vi "Triangular PDF.vi"(8 "xmax":dbl=1.0, 9 "xmode":dbl=nan, 10 "xmin":dbl, 11 "x":dbl=0.5) -> (0 "error":i32, 3 "pdf(x)":dbl=2.0)   [LabVIEW 2018, in "NI_Gmath.lvlib"]
doc: "Computes the continuous probability density function (PDF) of various distributions. You must manually select the polymorphic instance to use."
uses:
  NI_Gmath.lvlib
  st_error_code.ctl
panel:
  # "Triangular PDF"
  # "NaN maps to \n(xmax-xmin)/2"
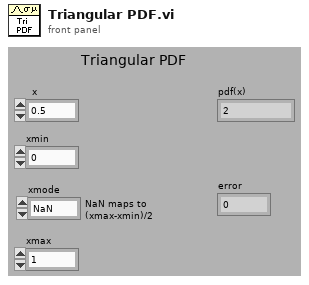
[diagram p1: front panel]
types:
  T1 = typedef "NI_Gmath.lvlib/st_error_code.ctl" = i32
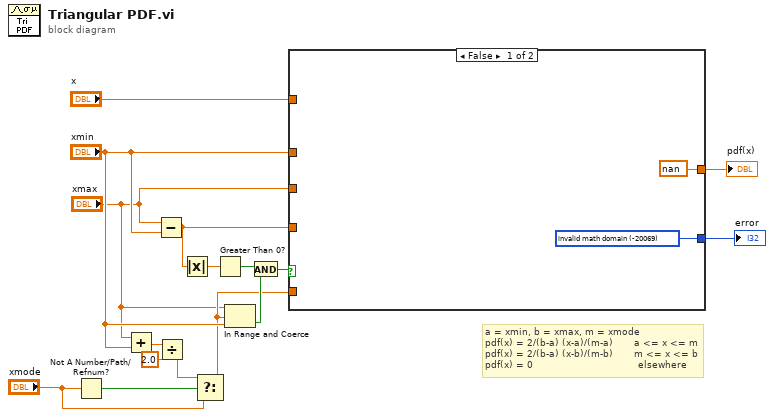
[diagram p0: block diagram]
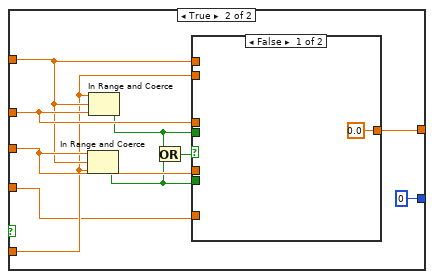
[diagram p2: hidden frame]
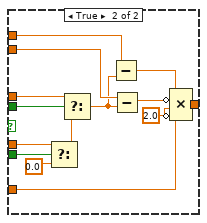
[diagram p3: hidden frame]
diagram:
  # "a = xmin, b = xmax, m = xmode\npdf(x) = 2/(b-a) (x-a)/(m-a)       a <= x <= m\npdf(x) = 2/(b-a) (x-b)/(m-b)       m <= x <= b\npdf(x) = 0                                   elsewhere"
  n1 = Not A Number/Path/Refnum?(number/path/refnum="xmode") -> (NaN/Path/Refnum?=w5:bool)
  n2 = Add(x="xmax", y="xmin") -> (x+y=w8:dbl)
  n3 = Subtract(x="xmax", y="xmin") -> (x-y=w10:dbl)
  n4 = Divide(x=w8, y=2.0) -> (x/y=w6:dbl)
  n5 = Absolute Value(x=w10) -> (abs(x)=w15:dbl)
  n6 = Select(t=w6, s=w5, f="xmode") -> (s? t:f=w2:dbl)
  n7 = Greater Than 0?(x=w15) -> (x > 0?=w12:bool)
  n8 = In Range and Coerce(upper limit="xmax", x=w2, lower limit="xmin") -> (In Range?=w3:bool)  [unwired: 1 out]
  n9 = And(x=w12, y=w3) -> (x .and. y?=w11:bool)
  n10 = case shown="False" w11 {
    tunnel: "x" -> [_ w25]
    tunnel: "xmin" -> [_ w27]
    tunnel: w10 -> [_ w23]
    tunnel: [nan w22] -> w14
    tunnel: [w17 0] -> w13
    tunnel: w2 -> [_ w24]
    tunnel: "xmax" -> [_ w26]
    frame False {
      w17 = T1 -20069 items=["invalid math domain"=-20069, "Fourier interpolation size m >= n"=-20070, "empty array"=-20003] ("stat interp error code")
    }
    frame True {
      n11 = In Range and Coerce(upper limit=w26, x=w25, lower limit=w24) -> (In Range?=w20:bool)  [unwired: 1 out]
      n12 = In Range and Coerce(upper limit=w24, x=w25, lower limit=w27) -> (In Range?=w21:bool)  [unwired: 1 out]
      n13 = Or(x=w21, y=w20) -> (x .or. y?=w19:bool)
      n14 = case shown="False" w19 {
        tunnel: w21 -> [_ w43]
        tunnel: w27 -> [_ w42]
        tunnel: w20 -> [_ w41]
        tunnel: w26 -> [_ w40]
        tunnel: w25 -> [_ w37]
        tunnel: w24 -> [_ w36]
        tunnel: w23 -> [_ w31]
        tunnel: [0.0 w30] -> w22
        frame False {
        }
        frame True {
          n15 = Select(t=w40, s=w41, f=0.0) -> (s? t:f=w39:dbl)
          n16 = Select(t=w42, s=w43, f=w39) -> (s? t:f=w35:dbl)
          n17 = Subtract(x=w37, y=w35) -> (x-y=w34:dbl)
          n18 = Subtract(x=w36, y=w35) -> (x-y=w33:dbl)
          n19 = Compound Arithmetic op=MULTIPLY(w34, invert w33, 2.0, invert w31) -> (w30:dbl)
        }
      }
    }
  }
  "pdf(x)" <- w14
  "error" <- w13
